vi "Byte Count.vi"(9 "Bytes Available":i32, 10 "Bytes so far":i32, 11 "Bytes to Read":i32) -> (1 "Byte count":i32)   [LabVIEW 2020, in "PicoG-Core.lvlib" / "VisaResource.lvclass"]
uses:
  VisaResource.lvclass
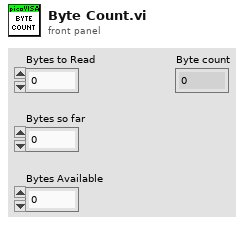
[diagram p1: front panel]
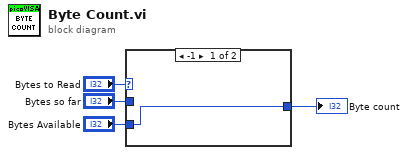
[diagram p0: block diagram]
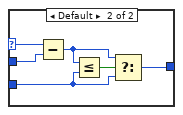
[diagram p2: hidden frame]
diagram:
  n1 = case shown="-1" "Bytes to Read" {
    selector: "Bytes to Read" -> [_ w10]
    tunnel: "Bytes so far" -> [_ w11]
    tunnel: "Bytes Available" -> [w5 w7]
    tunnel: [w5 w6] -> w1
    frame -1 {
    }
    frame Default {
      n2 = Subtract(x=w10, y=w11) -> (x-y=w8:i32)
      n3 = Less Or Equal?(x=w8, y=w7) -> (x <= y?=w9:bool)
      n4 = Select(t=w8, s=w9, f=w7) -> (s? t:f=w6:i32)
    }
  }
  "Byte count" <- w1
